vi "Joystick and Camera SHIH question.vi"(4 "right Std dev":dbl[](array[numeric]), 5 "right final out":dbl[](array[numeric]) format="%#_8g", 6 "left Std dev":dbl[](array[numeric]), 7 "left final out":dbl[](array[numeric]) format="%#_8g", 8 "down Std dev":dbl[](array[numeric]), 9 "down final out":dbl[](array[numeric]) format="%#_8g", 10 "up Std dev":dbl[](array[numeric]), 11 "up final out":dbl[](array[numeric]) format="%#_8g") -> (0 "Y 1":dbl[](array[numeric]) format="%#_8g", 1 "Y 2":dbl[](array[numeric]) format="%#_8g", 2 "X 2":dbl[](array[numeric]) format="%#_8g", 3 "X 1":dbl[](array[numeric]) format="%#_8g")   [LabVIEW 2016]
panel:
  out "left - right":dbl[](array[numeric]) format="%#_8g"
  out "up - down":dbl[](array[numeric]) format="%#_8g"
  in  "right used":bool=TRUE
  in  "left used":bool=TRUE
  in  "down used":bool=TRUE
  in  "up used":bool=TRUE
  in  "stop":bool
  # "Double true == Double false"
  # "For X axis"
  # "For Y axis"
  # "up"
  # "down"
  # "left"
  # "right"
  # "X sted dev"
  # "X sted dev"
  # "X sted dev"
  # "X sted dev"
  # "Y Std dev"
  # "Y Std dev"
  # "Y Std dev"
  # "Y Std dev"
  # "radius"
  # "radius"
  # "radius"
  # "radius"
  # "radius std dev"
  # "radius std dev"
  # "radius std dev"
  # "radius std dev"
  # "final out"
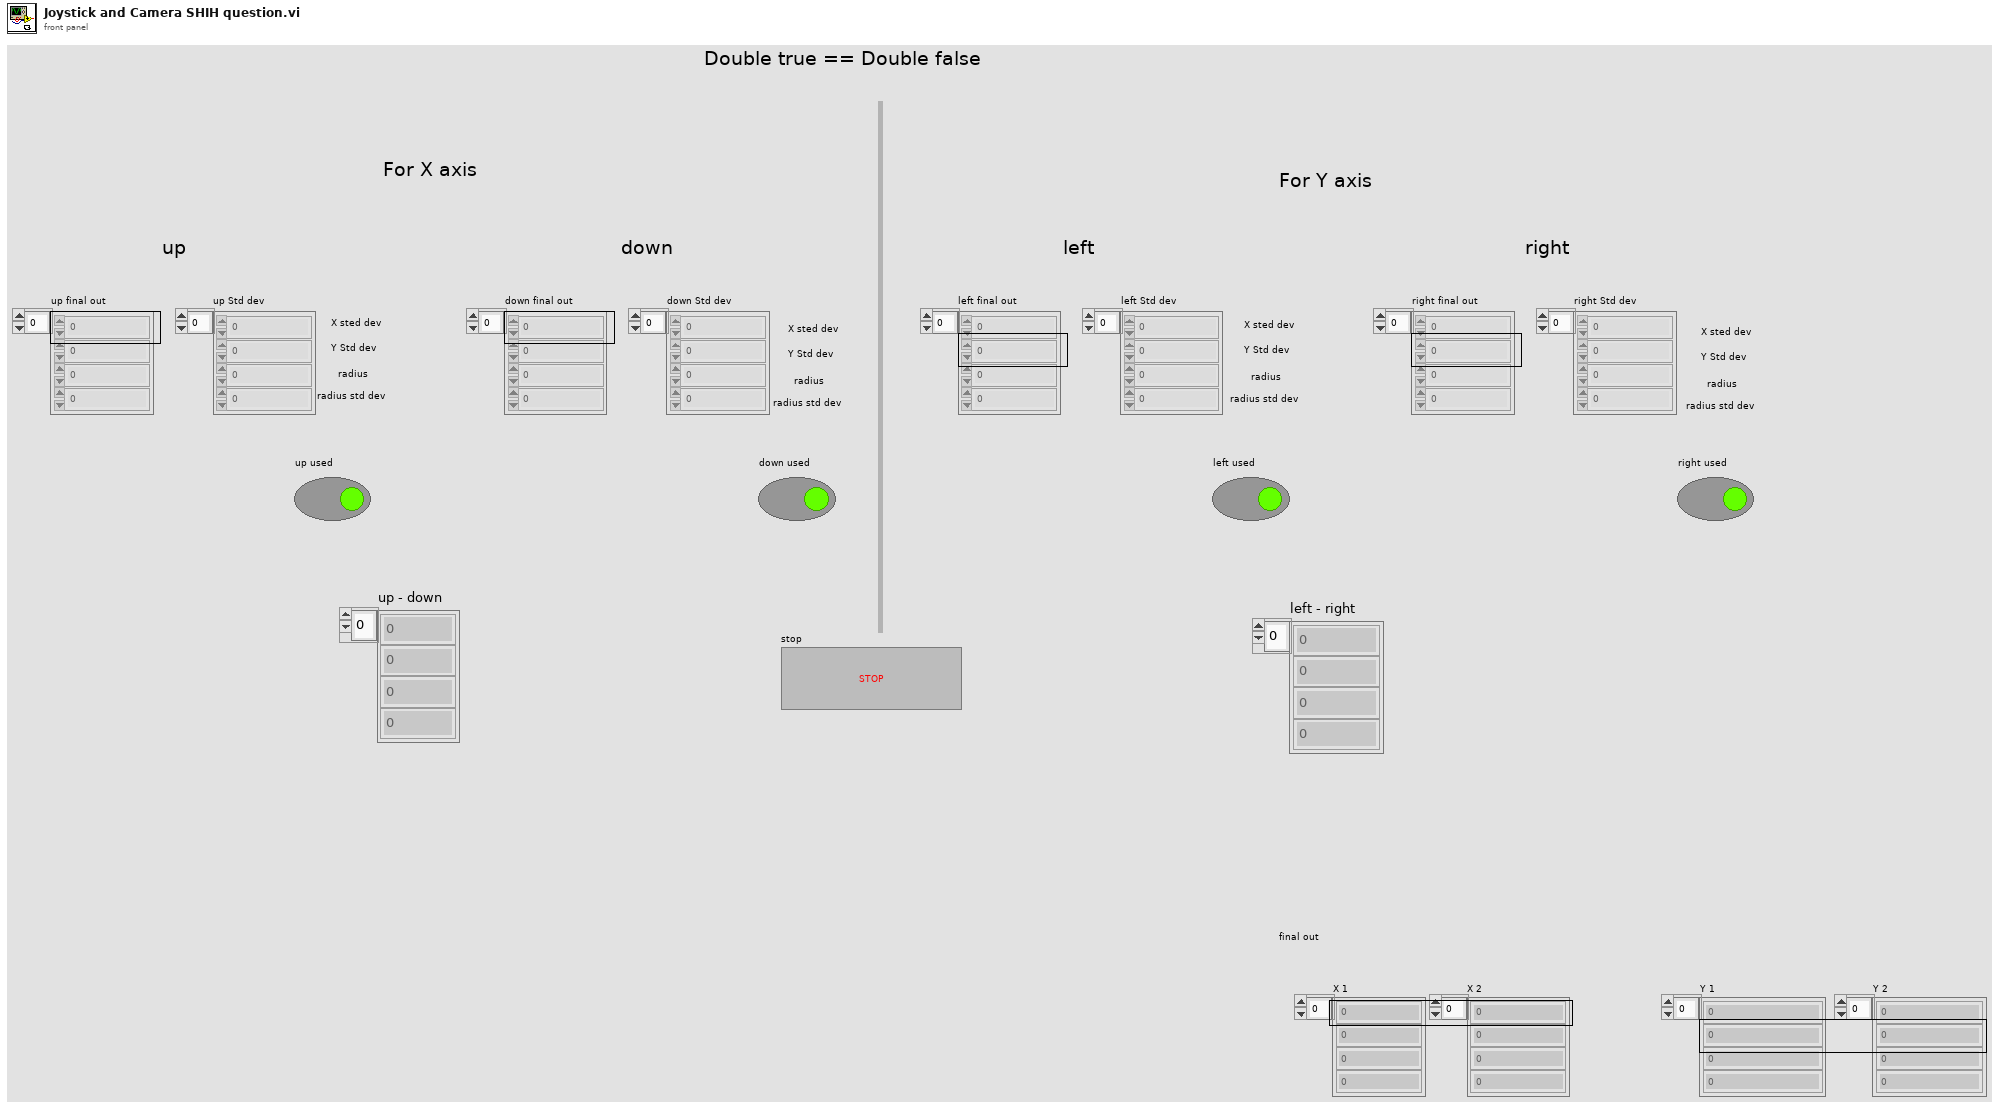
[diagram p1: front panel]
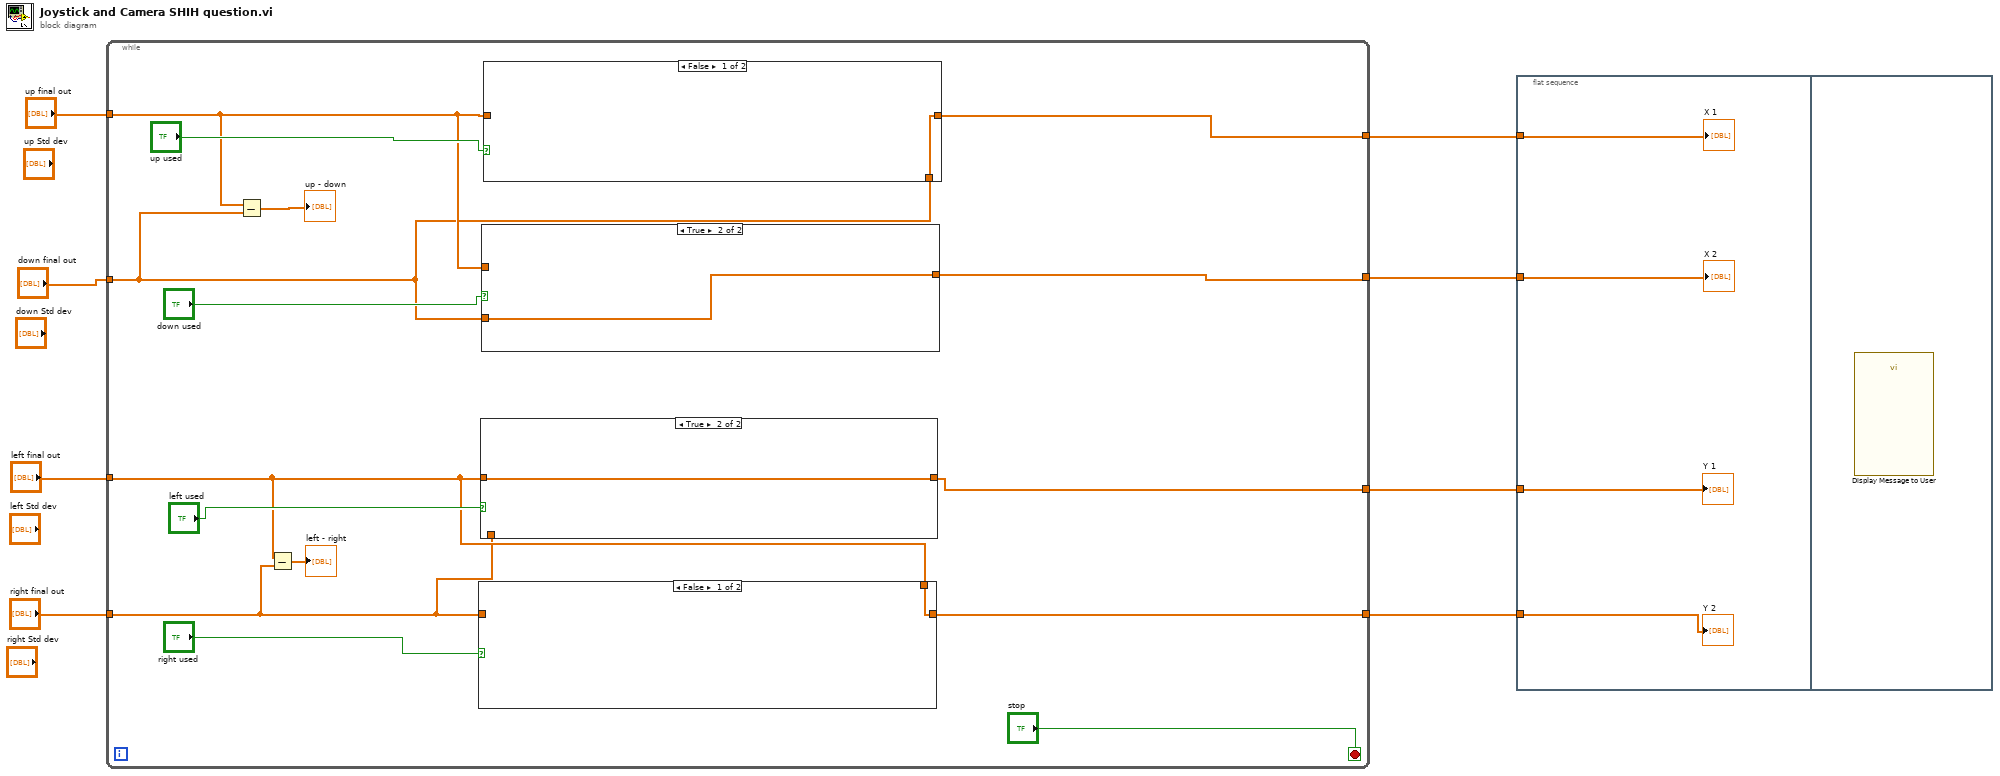
[diagram p0: block diagram]
diagram:
  n1 = while {
    tunnel: "up final out" -> [w14]
    tunnel: [w18] -> w7
    tunnel: "down final out" -> [w13]
    tunnel: [w17] -> w5
    tunnel: "left final out" -> [w11]
    tunnel: [w16] -> w3
    tunnel: "right final out" -> [w10]
    tunnel: [w15] -> w1
    stop <- "stop" stop-if-true
    n2 = Subtract(x=w14, y=w13) -> (x-y=→"up - down":dbl[])
    n3 = Subtract(x=w11, y=w10) -> (x-y=→"left - right":dbl[])
    n4 = case shown="False" "right used" {
      tunnel: w10 -> [_ w25]
      tunnel: [w24 w25] -> w15
      tunnel: w11 -> [w24 _]
      frame False {
      }
      frame True {
      }
    }
    n5 = case shown="True" "left used" {
      tunnel: w11 -> [_ w27]
      tunnel: [w26 w27] -> w16
      tunnel: w10 -> [w26 _]
      frame False {
      }
      frame True {
      }
    }
    n6 = case shown="True" "down used" {
      tunnel: [w28 w29] -> w17
      tunnel: w13 -> [_ w29]
      tunnel: w14 -> [w28 _]
      frame False {
      }
      frame True {
      }
    }
    n7 = case shown="False" "up used" {
      tunnel: w14 -> [_ w31]
      tunnel: [w30 w31] -> w18
      tunnel: w13 -> [w30 _]
      frame False {
      }
      frame True {
      }
    }
  }
  n8 = flat-sequence {
    tunnel: w7 -> [w35]
    tunnel: w5 -> [w34]
    tunnel: w3 -> [w33]
    tunnel: w1 -> [w32]
    frame #0 {
      "X 1" <- w35
      "X 2" <- w34
      "Y 1" <- w33
      "Y 2" <- w32
    }
    frame #1 {
      n9 = call "Display Message to User"() -> ()  [unwired: 10 in, 2 out]
    }
  }
